vi "Get SMO Address.vi"(8 "error in (no error)":errorcluster, 11 "Inst.TC in":refnum<class "Inst.TC.lvclass">) -> (0 "error out":errorcluster, 2 "SMO Address":string, 3 "Inst.TC out":refnum<class "Inst.TC.lvclass">)   [LabVIEW 2019, in "Inst.TC.lvclass"]
uses:
  Inst.TC.lvclass
  C:/Program Files (x86)/National Instruments/LabVIEW 2019/user.lib/LevyLab/Instrument Framework/SMOs/Instrument/Instrument.lvclass
  Inst.TC.lvclass/Inst.TC.ctl
  <userlib>/LevyLab/Instrument Framework/Instrument Types/VSource/Instrument.VSource.lvclass
  <userlib>/LevyLab/Instrument Framework/SMOs/Instrument/Instrument.lvclass
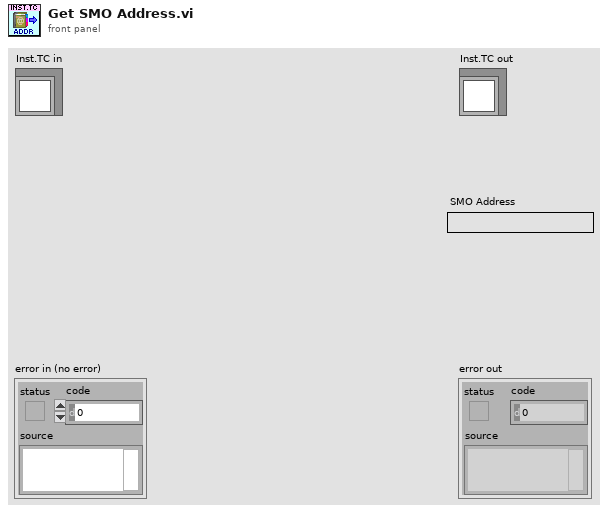
[diagram p1: front panel]
types:
  T1 = typedef "Inst.TC.lvclass/Inst.TC.Type--Enum.ctl" = enum16{"CF.TC", "CF.TC.Z", "CF.FP", "MNK.TC", "MNK.TC.Z", "MNK.FP"}
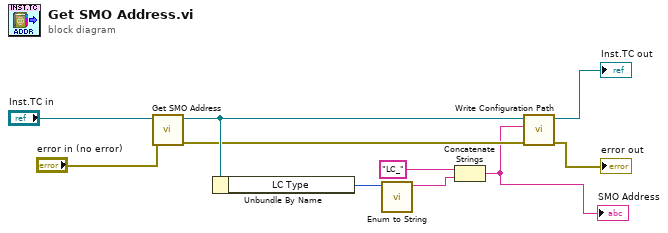
[diagram p0: block diagram]
diagram:
  n1 = call-parent "Get SMO Address.vi"("error in (no error)"="error in (no error)", "Instrument in"="Inst.TC in") -> ("error out"=w3:errorcluster, "Instrument out"=w5:refnum<class "Inst.TC.lvclass">)  [unwired: 7 in, 1 out]
  n2 = Unbundle By Name(w5) -> ("LC Type"=w7:T1)
  n3 = call <userlib>:"Enum to String.vi"("Command"=w7) -> ("Command"=w6:string)  [unwired: 9 in, 1 out]
  n4 = Concatenate Strings("LC_" ("SMO Name"), w6) -> (w2:string)
  "SMO Address" <- w2
  n5 = call <userlib>:"Write Configuration Path.vi"("error in (no error)"=w3, "name or relative path"=w2, "Instrument in"=w5) -> ("error out"=→"error out":errorcluster, "Instrument out"=→"Inst.TC out":refnum<class "Inst.TC.lvclass">)  [unwired: 7 in]
